vi "temperature_plotting.vi"() -> ()   [LabVIEW 2021]
panel:
  out "Waveform Graph":dbl[](graph)
  out "Waveform Chart":dbl(graph)
  in  "?":bool
  in  "On/Off":bool
  out "Temperature (F/C)":dbl(slide) scale=0.0..100.0
  in  "Temperature (F)":dbl(slide) scale=0.0..100.0
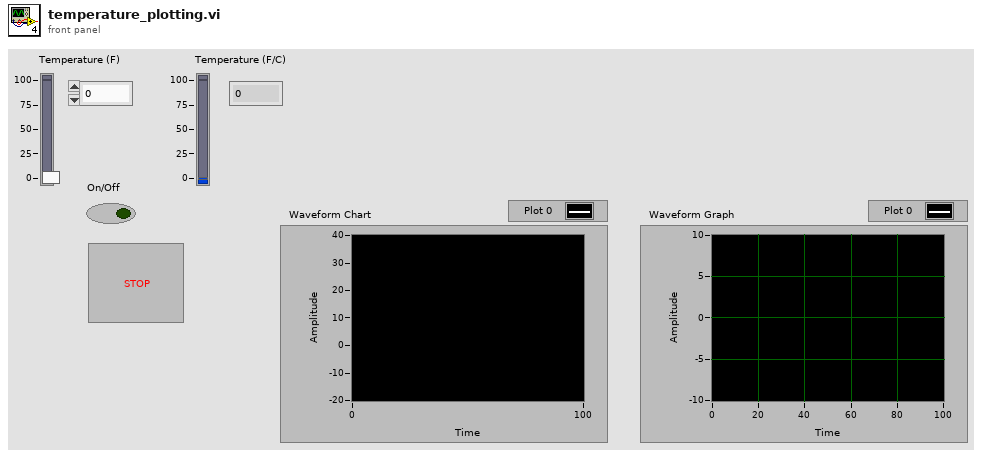
[diagram p1: front panel]
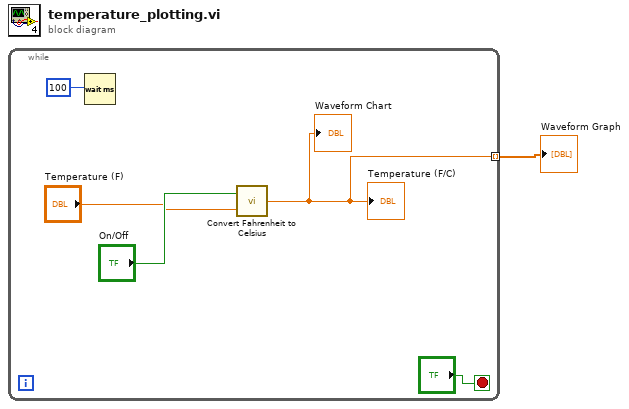
[diagram p0: block diagram]
diagram:
  n1 = while {
    tunnel: [w2] -> w1 mode=indexing
    stop <- "?" stop-if-true
    n2 = Wait (ms)(milliseconds to wait=100) -> ()  [unwired: 1 out]
    n3 = call "Convert Fahrenheit to Celsius.vi"("Fahrenheit"="Temperature (F)", "Boolean"="On/Off") -> ("Celsius"=w2:dbl)
    "Temperature (F/C)" <- w2
    "Waveform Chart" <- w2
  }
  "Waveform Graph" <- w1
